vi "Main_Host.vi"() -> ()   [LabVIEW 2014]
uses:
  RT/Controls/RT Stream Data.ctl
  UI Stop.vi
panel:
  in  "Exit":bool
  out "Faults":string="No Fault"
  out "System Status":string="Idle"
  in  "IP Address":string="169.254.125.17"
  in  "Tab Control":enum32{"Main", "System Monitoring"}(tab)
  in  "Manual":bool
  in  "pH Override":dbl=4.0
  in  "Temperature Override":dbl=20.0
  out "pH":dbl[](graph)
  out "Temperature":dbl[](graph)
  out "RAM %":dbl=22.359227203287748
  out "CPU %":dbl=28.85836037131932
  out "CPU %":dbl(graph)=28.85836037131932
  out "Memory (RAM) %":dbl(graph)=22.359227203287748
  out "Connected?":bool
  in  "Connect":bool
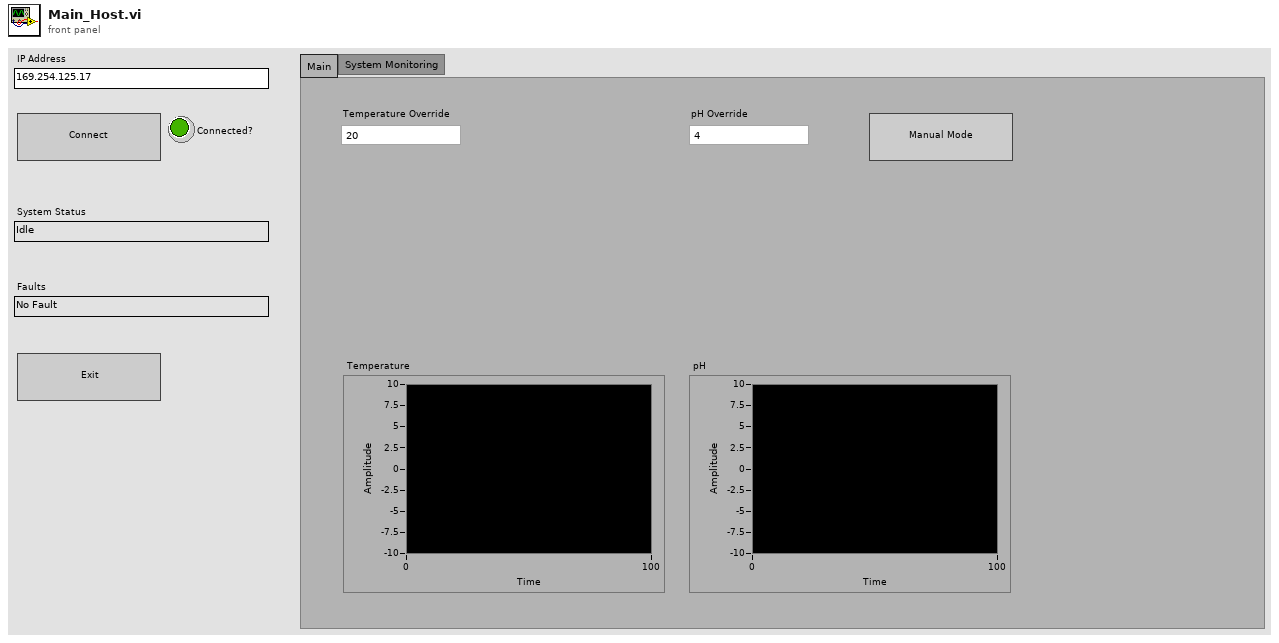
[diagram p1: front panel]
types:
  T1 = typedef "RT Stream Data.ctl" = cluster{"Temp Data":dbl[], "pH Data":dbl[]}
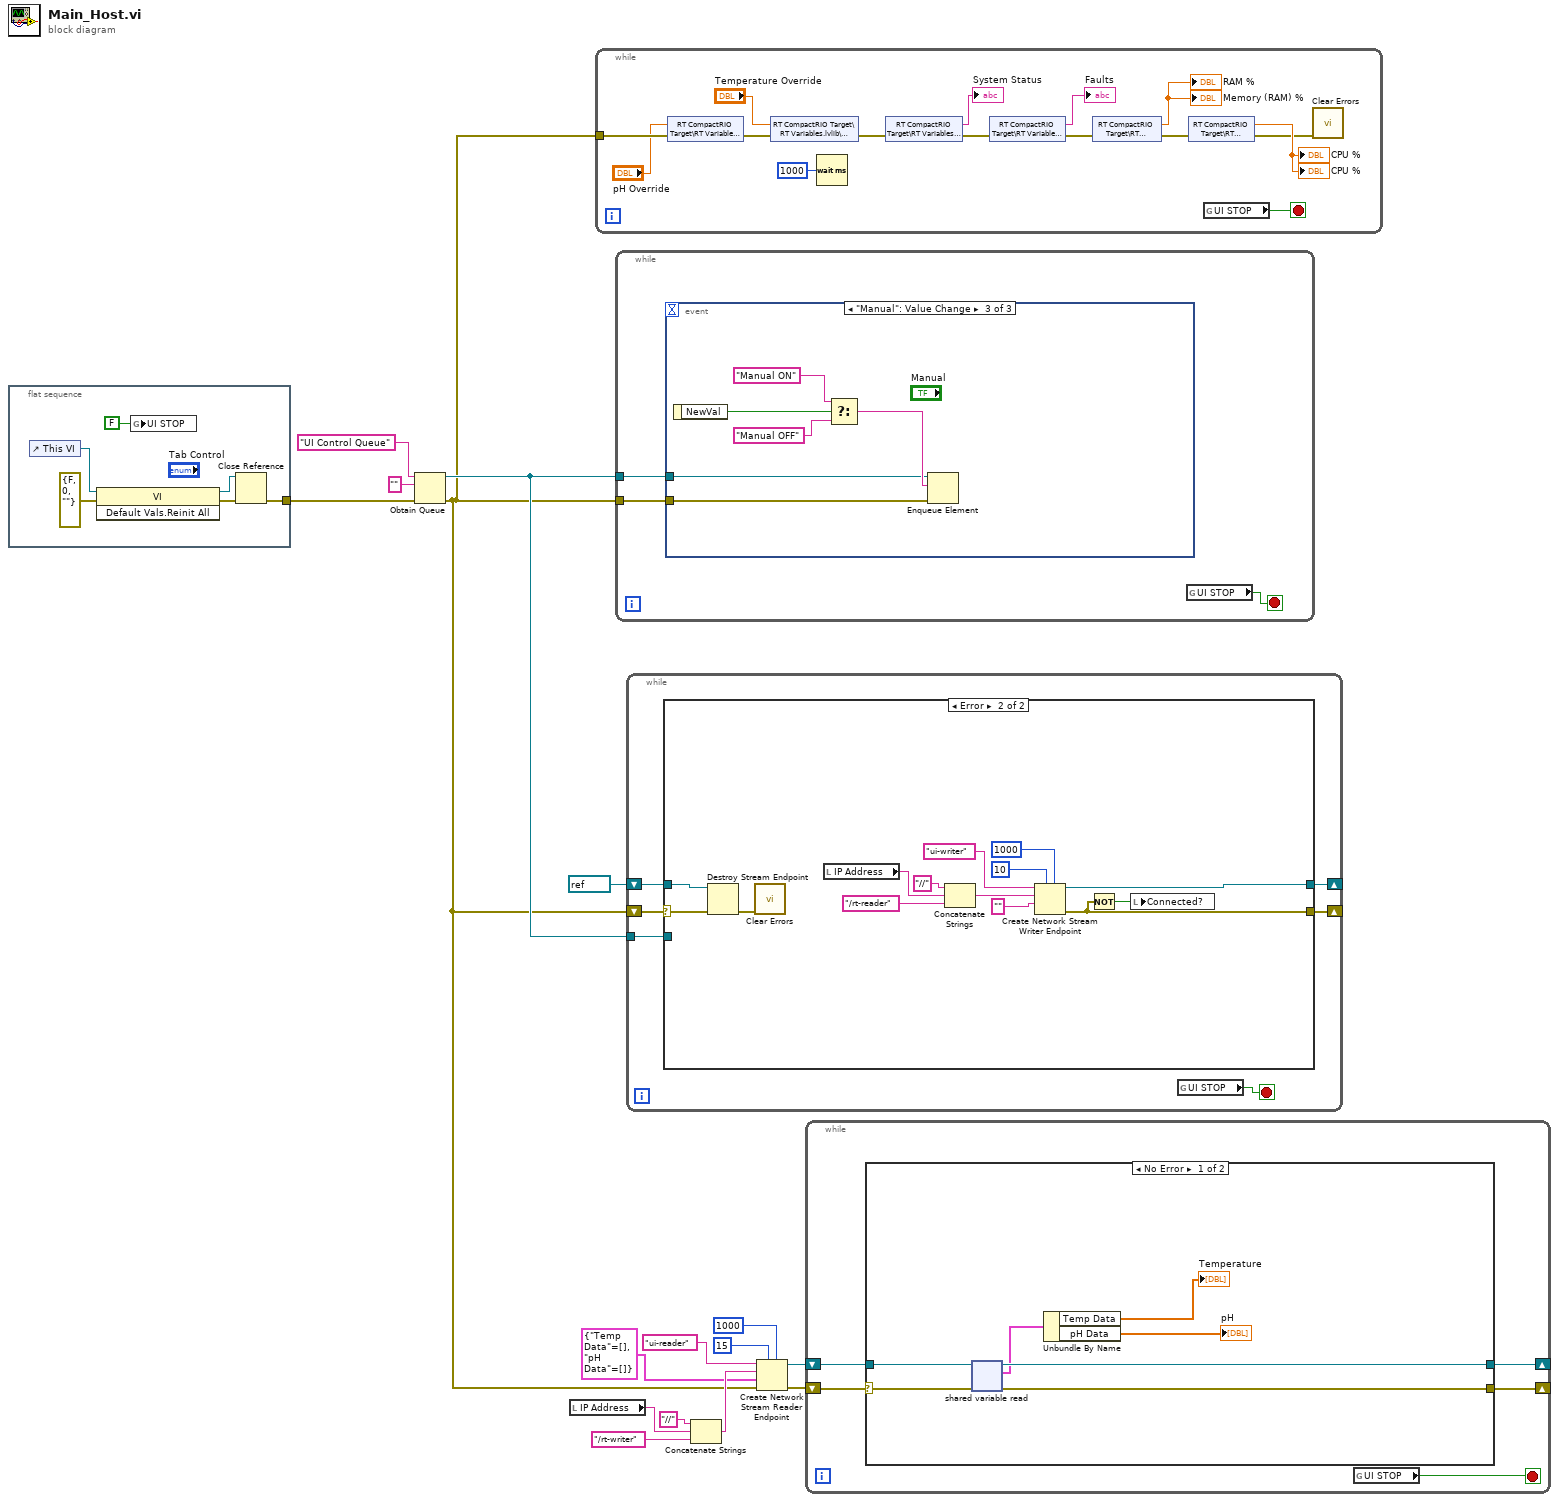
[diagram p0: block diagram]
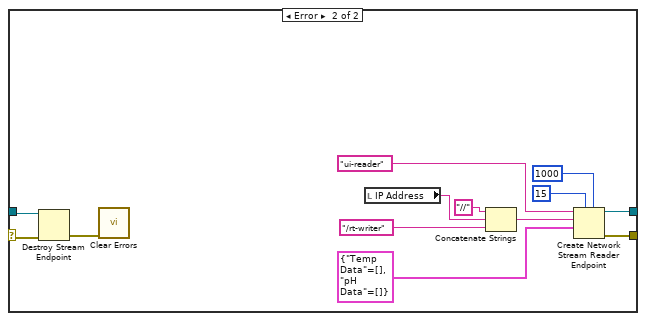
[diagram p2: hidden frame]
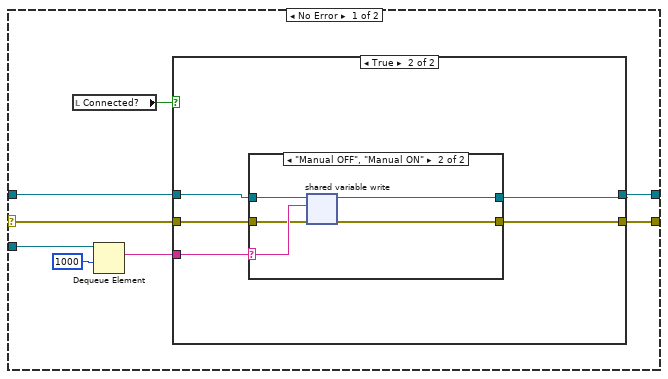
[diagram p3: hidden frame]
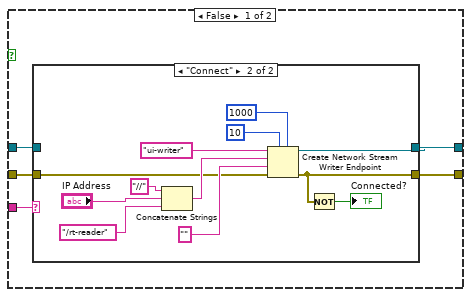
[diagram p4: hidden frame]
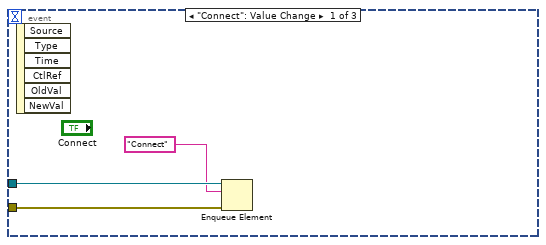
[diagram p7: hidden frame]
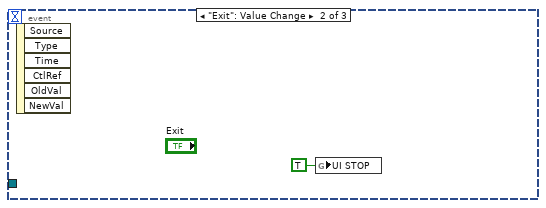
[diagram p8: hidden frame]
diagram:
  n1 = flat-sequence {
    tunnel: [w18] -> w15
    frame #0 {
      n2 = control-ref of="This VI"() -> (w20:refnum<vi>)
      n3 = invoke class="VI" method="Default Vals.Reinit All"(reference=w20, error in=errorcluster {"status"=FALSE, "code"=0, "source"=""} ("error in (no error)")) -> (reference out=w17:refnum<vi>, error out=w21:errorcluster)  [unwired: 1 in, 1 out]
      n4 = global write "UI Stop.vi" "UI STOP"(FALSE ("UI STOP")) -> ()
      n5 = Close Reference(reference=w17, error in (no error)=w21) -> (error out=w18:errorcluster)
    }
  }
  n6 = Obtain Queue(name (unnamed)="UI Control Queue", element data type="", error in (no error)=w15) -> (queue out=w14:refnum<queue>, error out=w1:errorcluster)  [unwired: 2 in, 1 out]
  n7 = local read "IP Address"() -> (w5:string)
  n8 = while {
    tunnel: w1 -> [w30]
    stop <- w37 stop-if-true
    n9 = shared-variable "RT CompactRIO Target\\RT Variables.lvlib\\pHOV"("pH Override", error in=w30) -> (error out=w36:errorcluster)
    n10 = shared-variable "RT CompactRIO Target\\RT Variables.lvlib\\TempOV"("Temperature Override", error in=w36) -> (error out=w35:errorcluster)
    n11 = Wait (ms)(milliseconds to wait=u32 1000) -> ()  [unwired: 1 out]
    n12 = shared-variable "RT CompactRIO Target\\RT Variables.lvlib\\Status"(error in=w35) -> (→"System Status":string, error out=w34:errorcluster)
    n13 = shared-variable "RT CompactRIO Target\\RT Variables.lvlib\\Faults"(error in=w34) -> (→"Faults":string, error out=w33:errorcluster)
    n14 = shared-variable "RT CompactRIO Target\\RT Variables.lvlib\\RAM"(error in=w33) -> (→"Memory (RAM) %" →"RAM %":dbl, error out=w32:errorcluster)
    n15 = shared-variable "RT CompactRIO Target\\RT Variables.lvlib\\CPU"(error in=w32) -> (→"CPU %" →"CPU %":dbl, error out=w23:errorcluster)
    n16 = global read "UI Stop.vi" "UI STOP"() -> (w37:bool)
    n17 = call <vilib>:"Clear Errors.vi"("error in (no error)"=w23) -> ()  [unwired: 5 in, 2 out]
  }
  n18 = while {
    tunnel: w14 -> [w39]
    tunnel: w1 -> [w38]
    stop <- w40 stop-if-true
    n19 = event shown="[2] \"Manual\": Value Change" {
      selector: _ -> [_ _ _]
      dyn-events: _ -> [_ _ _]
      timeout: _ -> [_ _ _]
      tunnel: w39 -> [w43 _ w46]
      tunnel: w38 -> [w42 _ w45]
      event "Connect": Value Change {
        n20 = event-data() -> ()  [unwired: 1 in, 6 out]
        n21 = Enqueue Element(queue=w43, element="Connect", error in (no error)=w42) -> ()  [unwired: 1 in, 3 out]
      }
      event "Exit": Value Change {
        n22 = event-data() -> ()  [unwired: 1 in, 6 out]
        n23 = global write "UI Stop.vi" "UI STOP"(TRUE ("UI STOP")) -> ()
      }
      event "Manual": Value Change {
        n24 = event-data() -> ("NewVal"=w50:bool)  [unwired: 1 in]
        n25 = Select(t="Manual ON", s=w50, f="Manual OFF") -> (s? t:f=w47:string)
        n26 = Enqueue Element(queue=w46, element=w47, error in (no error)=w45) -> ()  [unwired: 1 in, 3 out]
      }
    }
    n27 = global read "UI Stop.vi" "UI STOP"() -> (w40:bool)
  }
  n28 = while {
    tunnel: w14 -> [w54]
    shift-right: [w53] -> _
    shift-left: w1 -> [w55]
    shift-right: [w52] -> _
    shift-left: refnum<k21> refnum ("writer name") -> [w51]
    stop <- w56 stop-if-true
    n29 = case shown="Error" w55 {
      selector: w55 -> [w60 w108]
      tunnel: w54 -> [w62 _]
      tunnel: [w59 w96] -> w53
      tunnel: [w58 w97] -> w52
      tunnel: w51 -> [w57 w109]
      frame No Error {
        n30 = local read "Connected?"() -> (w64:bool)
        n31 = Dequeue Element(queue=w62, timeout in ms (-1)=1000) -> (element=w61:string)  [unwired: 1 in, 3 out]
        n32 = case shown="True" w64 {
          tunnel: w61 -> [w69 w88]
          tunnel: w60 -> [w68 w84]
          tunnel: [w67 w85] -> w59
          tunnel: [w66 w86] -> w58
          tunnel: w57 -> [w65 w87]
          frame False {
            n33 = case shown="\"Connect\"" w69 {
              tunnel: w68 -> [w70 w75]
              tunnel: [w70 w73] -> w67
              tunnel: [w71 w74] -> w66
              tunnel: w65 -> [w71 _]
              frame "False", Default {
              }
              frame "Connect" {
                n34 = Concatenate Strings("//" ("string"), "IP Address", "/rt-reader" ("string")) -> (w80:string)
                n35 = Create Network Stream Writer Endpoint(5:1000 ("timeout in ms (-1)"), 7:10 ("writer buffer size"), 8:w75, 9:"", 10:w80, 11:"ui-writer" ("writer name")) -> (0:w73:errorcluster, 3:w74:refnum<k21>)  [unwired: 1 in]
                n36 = Not(x=w73) -> (.not. x?=→"Connected?":bool)
              }
            }
          }
          frame True {
            n37 = case shown="\"Manual OFF\", \"Manual ON\"" w88 {
              selector: w88 -> [_ w95]
              tunnel: w87 -> [w90 w94]
              tunnel: [w90 w93] -> w86
              tunnel: [w89 w92] -> w85
              tunnel: w84 -> [w89 w91]
              frame "False", Default {
              }
              frame "Manual OFF", "Manual ON" {
                n38 = shared-variable-write(w94, w91, w95) -> (w93:refnum<k21>, w92:errorcluster)  [unwired: 1 in, 1 out]
              }
            }
          }
        }
      }
      frame Error {
        n39 = Destroy Stream Endpoint(8:w108, 11:w109) -> (0:w107:errorcluster)
        n40 = call <vilib>:"Clear Errors.vi"("error in (no error)"=w107) -> ()  [unwired: 5 in, 2 out]
        n41 = local read "IP Address"() -> (w106:string)
        n42 = Concatenate Strings("//" ("string"), w106, "/rt-reader" ("string")) -> (w103:string)
        n43 = Create Network Stream Writer Endpoint(5:1000 ("timeout in ms (-1)"), 7:10 ("writer buffer size"), 9:"", 10:w103, 11:"ui-writer" ("writer name")) -> (0:w96:errorcluster, 3:w97:refnum<k21>)  [unwired: 2 in]
        n44 = Not(x=w96) -> (.not. x?=w98:bool)
        n45 = local write "Connected?"(w98) -> ()
      }
    }
    n46 = global read "UI Stop.vi" "UI STOP"() -> (w56:bool)
  }
  n47 = Concatenate Strings("//" ("string"), w5, "/rt-writer" ("string")) -> (w8:string)
  n48 = Create Network Stream Reader Endpoint(5:1000 ("timeout in ms (-1)"), 7:15 ("writer buffer size"), 8:w1, 9:T1 {"Temp Data"=[], "pH Data"=[]} ("cluster"), 10:w8, 11:"ui-reader" ("writer name")) -> (0:w4:errorcluster, 3:w3:refnum<k21>)  [unwired: 1 in]
  n49 = while {
    shift-right: [w110] -> _
    shift-left: w4 -> [w113]
    shift-right: [w111] -> _
    shift-left: w3 -> [w112]
    stop <- w114 stop-if-true
    n50 = case shown="No Error" w113 {
      selector: w113 -> [w120 w124]
      tunnel: w112 -> [w121 w125]
      tunnel: [w119 w127] -> w111
      tunnel: [w118 w126] -> w110
      frame No Error {
        n51 = shared-variable-read(w121, w120) -> (w119:refnum<k21>, w118:errorcluster, w117:T1)  [unwired: 1 in, 1 out]
        n52 = Unbundle By Name(w117) -> ("Temp Data"=→"Temperature":dbl[], "pH Data"=→"pH":dbl[])
      }
      frame Error {
        n53 = Destroy Stream Endpoint(8:w124, 11:w125) -> (0:w123:errorcluster)
        n54 = call <vilib>:"Clear Errors.vi"("error in (no error)"=w123) -> ()  [unwired: 5 in, 2 out]
        n55 = local read "IP Address"() -> (w128:string)
        n56 = Concatenate Strings("//" ("string"), w128, "/rt-writer" ("string")) -> (w131:string)
        n57 = Create Network Stream Reader Endpoint(5:1000 ("timeout in ms (-1)"), 7:15 ("writer buffer size"), 9:T1 {"Temp Data"=[], "pH Data"=[]} ("cluster"), 10:w131, 11:"ui-reader" ("writer name")) -> (0:w126:errorcluster, 3:w127:refnum<k21>)  [unwired: 2 in]
      }
    }
    n58 = global read "UI Stop.vi" "UI STOP"() -> (w114:bool)
  }
